vi "WriteIconsTDMS.vi"() -> ()   [LabVIEW 2014]
uses:
  <vilib>/picture/picture.llb/imagedata.ctl
  <userlib>/_LAVACR/Scripting Tools/Scripting Tools.lvlib
panel:
  out "Array 5":i32[](array[numeric])
  out "Array 4":T1[](array[typedef])
  out "Array 3":T1[](array[typedef])
  out "Array 2":i32[](array[numeric])
  out "Array":picture[](array[picture])
  out "IconsFromFile":picture[](array[picture])
  in  "file path":path
  out "Class Hierarchy 2":string[][](array[string])
  out "Labels":string[](array[string])
  out "ClassName":string[](array[string])
  out "ClassName":string[](array[string])
  out "Class Hierarchy":string[][](array[string])
  out "Icons":picture[](array[picture])
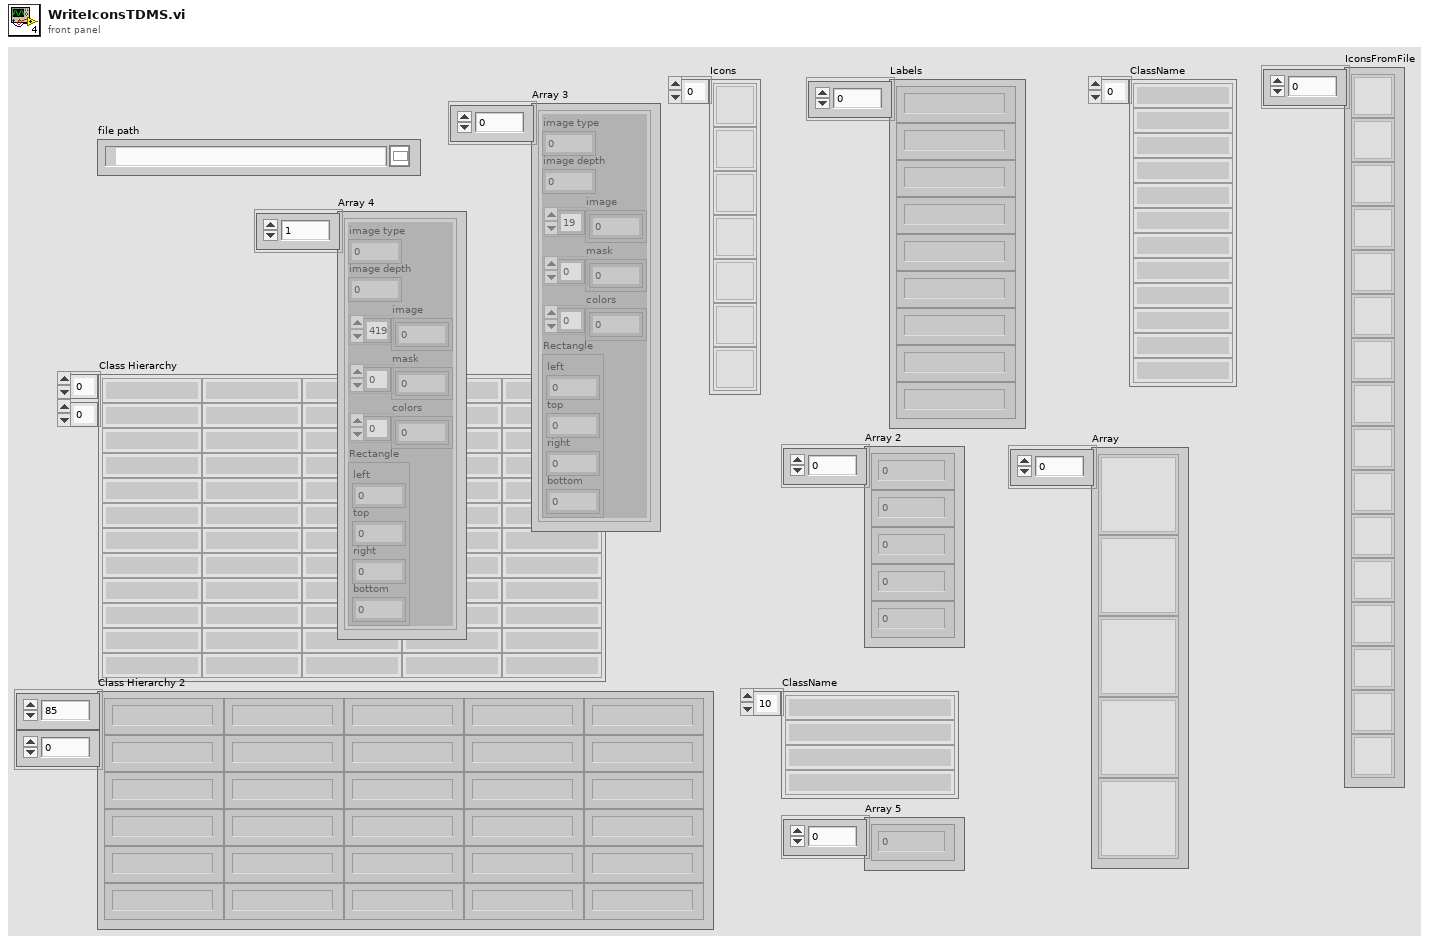
[diagram p1: front panel]
types:
  T1 = typedef "imagedata.ctl" = cluster{"image type":i32, "image depth":i32, "image":u8[], "mask":u8[], "colors":u32[], "Rectangle":cluster{"left":i16, "top":i16, "right":i16, "bottom":i16}}
  T2 = enum16{"open", "open or create", "create or replace", "create", "open (read-only)"}
  T3 = cluster{"left":i16, "top":i16, "right":i16, "bottom":i16}
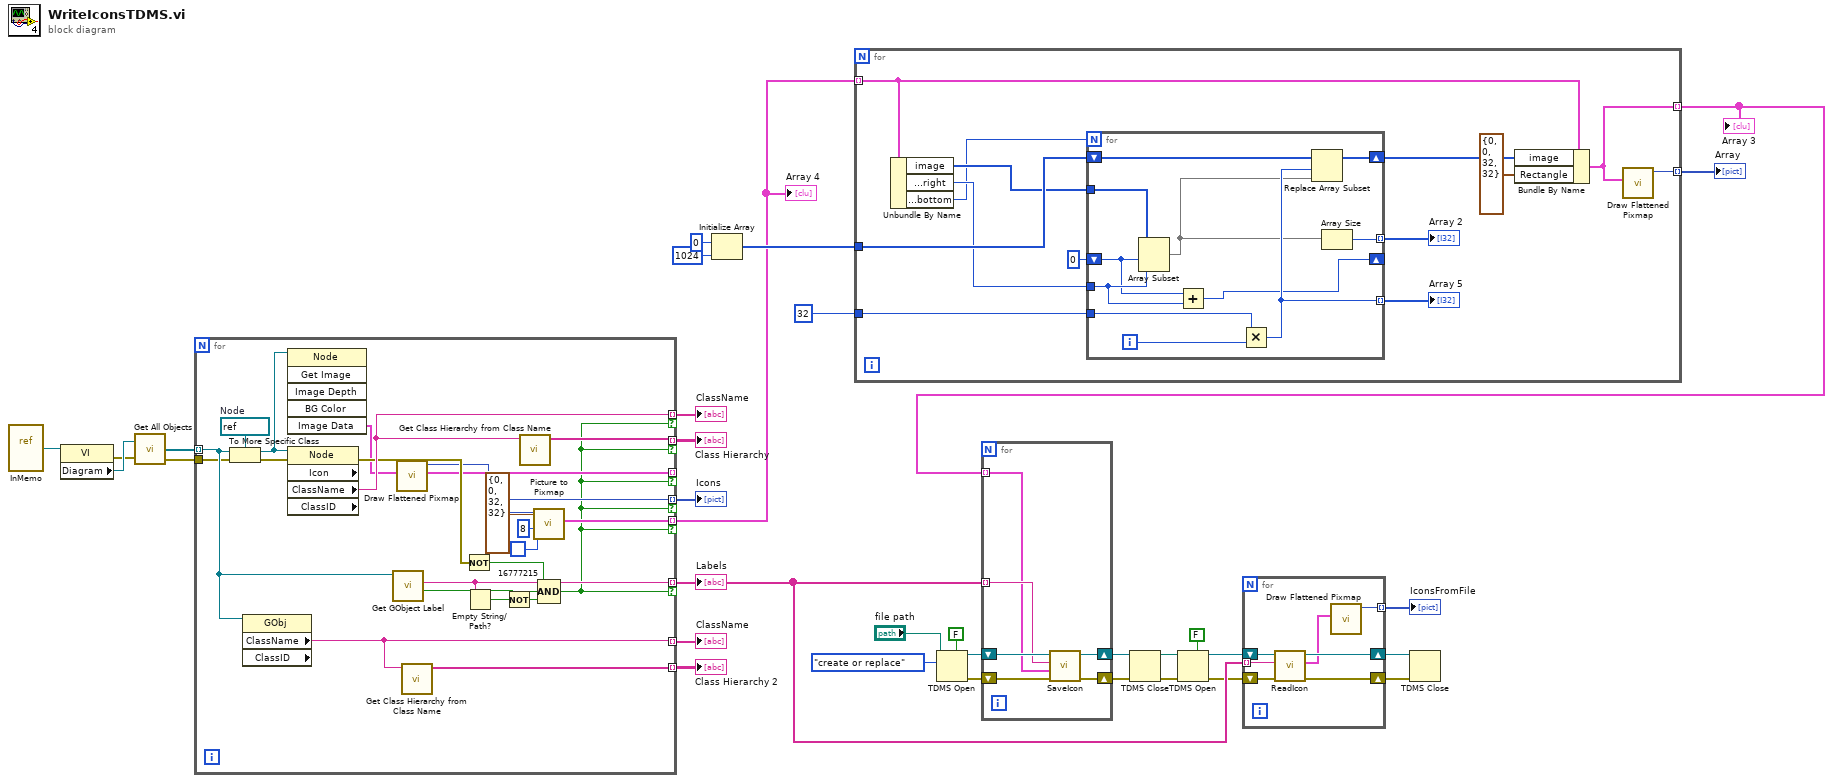
[diagram p0: block diagram]
diagram:
  n1 = vi-ref "InMemo.vi"() -> (w29:refnum<vi>)
  n2 = property class="VI"(reference=w29) -> (error out=w27:errorcluster, "Diagram"=w28:refnum<vi>)  [unwired: 1 in, 1 out]
  n3 = call <userlib>:"Get All Objects.vi"("Diagram In"=w28, "error in"=w27) -> ("All Objects"=w33:refnum<vi>[], "error out"=w26:errorcluster)  [unwired: 1 out]
  n4 = for {
    tunnel: w33 -> [w52] mode=indexing
    tunnel: [w39] -> w2 mode=indexing if=w36
    tunnel: [w54] -> w32 mode=indexing if=w36
    tunnel: [w53] -> w31 mode=indexing if=w36
    tunnel: [w44] -> w30 mode=indexing
    tunnel: [w51] -> w24 mode=indexing if=w36
    tunnel: [w43] -> w25 mode=indexing
    tunnel: w26 -> [w45]
    tunnel: [w40] -> _ mode=indexing if=w36
    tunnel: [w37] -> w1 mode=indexing if=w36
    w55 = refnum<vi> refnum  # Node
    n5 = To More Specific Class(target class=w55, reference=w52, error in=w45) -> (specific class reference=w41:refnum<vi>, error out=w42:errorcluster)
    n6 = property class="GObj" props=["ClassName", "ClassID"](reference=w52) -> ("ClassName"=w44:string)  [unwired: 1 in, 3 out]
    n7 = invoke class="Node" method="Get Image"(reference=w41) -> ("Image Data"=w40:T1)  [unwired: 5 in, 5 out]
    n8 = property class="Node" props=["Icon", "ClassName", "ClassID"](reference=w41, error in=w42) -> (error out=w47:errorcluster, "ClassName"=w53:string)  [unwired: 3 out]
    n9 = call <vilib>:"Get GObject Label.vi"("GObject"=w52) -> ("Object Has Label?"=w48:bool, "Object Label"=w51:string)  [unwired: 6 in, 3 out]
    n10 = call <vilib>:"Draw Flattened Pixmap.vi"("image data"=w40) -> ("new picture"=w39:picture)  [unwired: 8 in]
    n11 = call <vilib>:"Get Class Hierarchy from Class Name.vi"("Class Name"=w44) -> ("Class Hierarchy"=w43:string[])  [unwired: 9 in, 1 out]
    n12 = Not(x=w47) -> (.not. x?=w46:bool)
    n13 = Empty String/Path?(string/path=w51) -> (empty?=w50:bool)
    n14 = Not(x=w50) -> (.not. x?=w49:bool)
    n15 = call <vilib>:"Get Class Hierarchy from Class Name.vi"("Class Name"=w53) -> ("Class Hierarchy"=w54:string[])  [unwired: 9 in, 1 out]
    n16 = call <vilib>:"Picture to Pixmap.vi"("Background Color"=u32 16777215, "depth"=8, "rect"=T3 {"left"=0, "top"=0, "right"=32, "bottom"=32}, "picture"=w39) -> ("image data"=w37:T1)  [unwired: 6 in, 1 out]
    n17 = Compound Arithmetic op=AND(w46, w48, w49) -> (w36:bool)
  }
  "Icons" <- w2
  "Class Hierarchy" <- w32
  "ClassName" <- w31
  "ClassName" <- w30
  "Labels" <- w24
  "Class Hierarchy 2" <- w25
  "Array 4" <- w1
  n18 = Initialize Array(u8 0, 1024 ("dimension size")) -> (w20:u8[])
  n19 = for {
    tunnel: w1 -> [w68] mode=indexing
    tunnel: w20 -> [w67]
    tunnel: [w64] -> w21 mode=indexing
    tunnel: [w63] -> w4 mode=indexing
    tunnel: i16 32 ("Rectangle.right") -> [w58]
    n20 = Unbundle By Name(w68) -> ("image"=w66:u8[], "Rectangle.right"=w57:i16, "Rectangle.bottom"=w56:i16)
    n21 = for {
      N: w56 -> [_]
      tunnel: w66 -> [w74]
      shift-right: [w78] -> w65
      shift-left: w67 -> [w79]
      tunnel: w58 -> [w77]
      shift-right: [w69] -> _
      shift-left: 0 -> [w70]
      tunnel: w57 -> [w71]
      tunnel: [w76] -> w60 mode=indexing
      tunnel: [w75] -> w59 mode=indexing
      i -> [w72]
      n22 = Array Subset(array=w74, index=w70, length=w71) -> (w73:u8[])
      n23 = Add(x=w70, y=w71) -> (x+y=w69:i32)
      n24 = Multiply(x=w77, y=w72) -> (x*y=w75:i32)
      n25 = Replace Array Subset(array=w79, new element=w73, index=w75) -> (w78:u8[])
      n26 = Array Size(array=w73) -> (size(s)=w76:i32)
    }
    "Array 2" <- w60
    "Array 5" <- w59
    n27 = Bundle By Name(cluster=w68, "image"=w65, "Rectangle"=T3 {"left"=0, "top"=0, "right"=32, "bottom"=32}) -> (w63:T1)
    n28 = call <vilib>:"Draw Flattened Pixmap.vi"("image data"=w63) -> ("new picture"=w64:picture)  [unwired: 8 in]
  }
  "Array" <- w21
  "Array 3" <- w4
  n29 = TDMS Open(5:FALSE ("create index file? (T)"), 10:T2."create or replace" ("operation (0:open)"), 11:"file path") -> (0:w11:errorcluster, 3:w12:refnum<k34>)  [unwired: 4 in]
  n30 = for {
    tunnel: w24 -> [w82] mode=indexing
    shift-right: [w84] -> w9
    shift-left: w11 -> [w81]
    shift-right: [w83] -> w10
    shift-left: w12 -> [w85]
    tunnel: w4 -> [w80] mode=indexing
    n31 = call "SaveIcon.vi"("error in (no error)"=w81, "Icon"=w80, "Function"=w82, "TdmsIn"=w85) -> ("error out"=w84:errorcluster, "TdmsOuit"=w83:refnum<k34>)  [unwired: 6 in]
  }
  n32 = TDMS Close(8:w9, 11:w10) -> (0:w6:errorcluster, 3:w7:path)
  n33 = TDMS Open(5:FALSE ("create index file? (T)"), 8:w6, 11:w7) -> (0:w14:errorcluster, 3:w15:refnum<k34>)  [unwired: 4 in]
  n34 = for {
    shift-right: [w89] -> w8
    shift-left: w15 -> [w91]
    shift-right: [w92] -> w16
    shift-left: w14 -> [w90]
    tunnel: w24 -> [w88] mode=indexing
    tunnel: [w86] -> w5 mode=indexing
    n35 = call "ReadIcon.vi"("error in (no error)"=w90, "Function"=w88, "TdmsIn"=w91) -> ("error out"=w92:errorcluster, "Icon"=w87:T1, "TdmsOut"=w89:refnum<k34>)  [unwired: 6 in]
    n36 = call <vilib>:"Draw Flattened Pixmap.vi"("image data"=w87) -> ("new picture"=w86:picture)  [unwired: 8 in]
  }
  "IconsFromFile" <- w5
  n37 = TDMS Close(8:w16, 11:w8) -> ()  [unwired: 2 out]
